vi "to string.vi"(8 "error in":errorcluster, 11 "Modbus Slave configuration in":refnum<class "Modbus Slave configuration.lvclass">) -> (0 "error out":errorcluster, 1 "data":string, 2 "version":string, 3 "Modbus Slave configuration out":refnum<class "Modbus Slave configuration.lvclass">)   [LabVIEW 2013, in "Modbus Slave configuration.lvclass"]
doc: "Provides an interface for saving a module configuration to a file or other serialized data source. It is recommended that all children of this class store data in two sets--data required for its own initialization, and any data required for parent initialization--and that each implementation uses the <b>Call Parent Method</b> primitive to serialize parent information.Platypus Framework 1.0.1.65\nNI Systems Engineering - National Instruments"
uses:
  Modbus Slave configuration.lvclass
  <vilib>/NI/Tag Bus Module Framework/module configuration/TBM module configuration.lvclass
  Modbus Slave configuration.lvclass/Modbus Slave configuration.ctl
  module channel/Modbus Module Channel.lvclass
  <vilib>/NI/Tag Bus Module Framework/root configuration/unwrap data.vi
  <vilib>/NI/Tag Bus Module Framework/root configuration/TBM configuration.lvclass
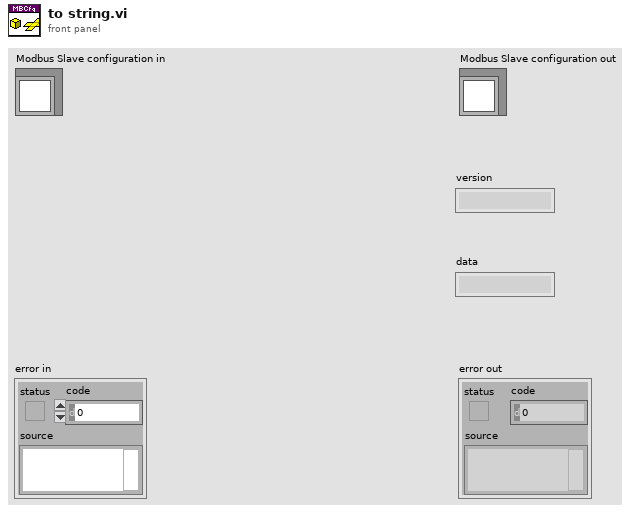
[diagram p1: front panel]
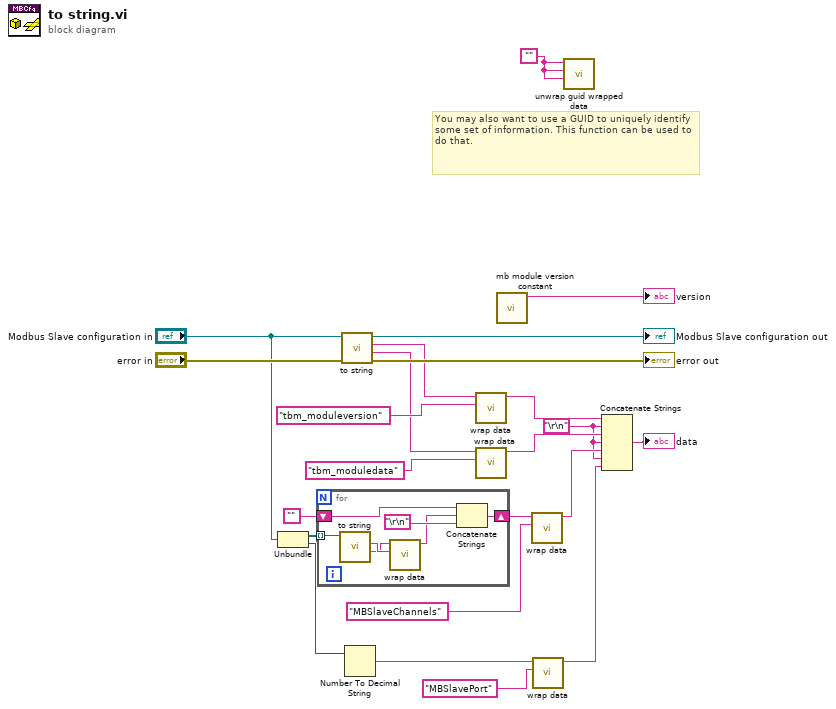
[diagram p0: block diagram]
diagram:
  w5 = "\r\n"
  w14 = ""
  # "You may also want to use a GUID to uniquely identify some set of information. This function can be used to do that."
  n1 = Unbundle("Modbus Slave configuration in") -> (w9:refnum<class "Modbus Module Channel.lvclass">[], w3:u16)
  n2 = for {
    tunnel: w9 -> [w26] mode=indexing
    shift-right: [w29] -> w7
    shift-left: "" -> [w28]
    n3 = call-dynamic "to string.vi"("channel in"=w26) -> ("channel data"=w24:string, "identifier"=w25:string)  [unwired: 7 in, 2 out]
    n4 = call <vilib>:"wrap data.vi"("identifier"=w25, "data to wrap"=w24) -> ("wrapped data"=w27:string)  [unwired: 9 in]
    n5 = Concatenate Strings(w28, w27, "\r\n") -> (w29:string)
  }
  n6 = call-parent "to string.vi"("error in"="error in", "module configuration in"="Modbus Slave configuration in") -> ("error out"=→"error out":errorcluster, "data"=w15:string, "version"=w16:string, "module configuration out"=→"Modbus Slave configuration out":refnum<class "Modbus Slave configuration.lvclass">)  [unwired: 6 in]
  n7 = Number To Decimal String(number=w3) -> (decimal integer string=w2:string)  [unwired: 1 in]
  n8 = call <vilib>:"wrap data.vi"("identifier"="tbm_moduleversion" ("additional identifier"), "data to wrap"=w16) -> ("wrapped data"=w18:string)  [unwired: 9 in]
  n9 = call <vilib>:"wrap data.vi"("identifier"="tbm_moduledata" ("additional identifier"), "data to wrap"=w15) -> ("wrapped data"=w17:string)  [unwired: 9 in]
  n10 = call "mb module version constant.vi"() -> ("current version"=→"version":string)  [unwired: 11 in]
  n11 = call <vilib>:"wrap data.vi"("identifier"="MBSlaveChannels" ("additional identifier"), "data to wrap"=w7) -> ("wrapped data"=w11:string)  [unwired: 9 in]
  n12 = call <vilib>:"wrap data.vi"("identifier"="MBSlavePort" ("additional identifier"), "data to wrap"=w2) -> ("wrapped data"=w4:string)  [unwired: 9 in]
  n13 = call <vilib>:"unwrap guid wrapped data.vi"("identifier"=w14, "uuid"=w14, "data to unwrap"=w14) -> ()  [unwired: 7 in, 2 out]
  n14 = Concatenate Strings(w18, w5, w17, w5, w11, w5, w4) -> (→"data":string)
